vi "send samples.vi"(6 "sample valid before CFO":bool, 7 "use before CFO":bool, 8 "channels before CFO":T1, 9 "packet start":bool, 10 "sample valid after CFO":bool, 11 "channels after CFO":T1) -> ()   [LabVIEW 2020]
uses:
  <vilib>/rvi/interface/RandomDataEmulation/niFpgaRandomDataHandleErrors.vi
  <vilib>/rvi/DataTransferAndStorage/Container/XNode/niFpgaContainer.xnode
  <vilib>/rvi/interface/RandomDataEmulation/nirviRandomDataFpgaReadWriteTemplate.vi
panel:
  out "Imag":fxp<+/-,16,3>
  out "Real":fxp<+/-,16,3>
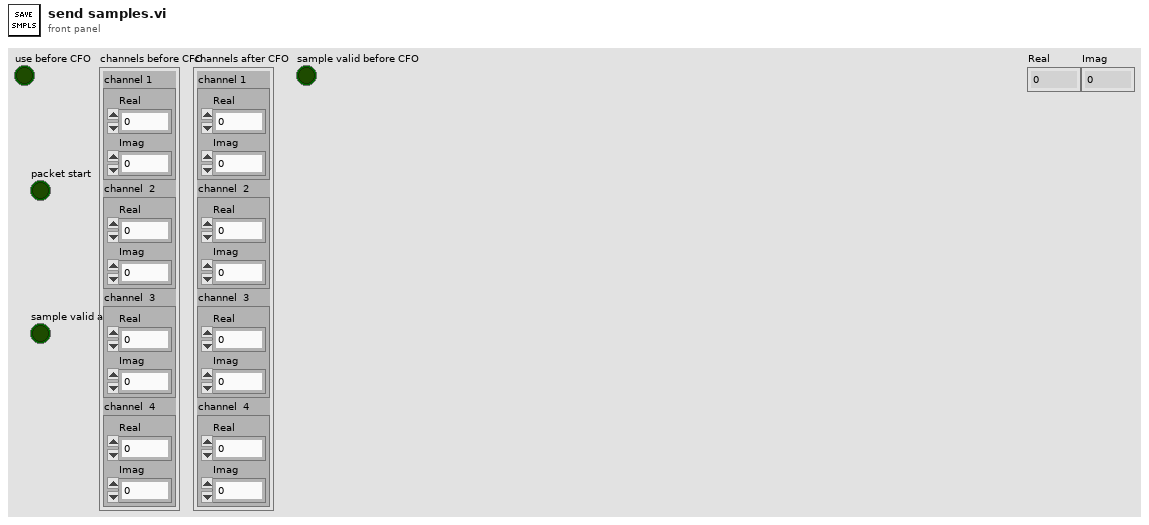
[diagram p1: front panel]
types:
  T1 = cluster{"channel 1 ":cluster{"Real":fxp<+/-,16,3>, "Imag":fxp<+/-,16,3>}, "channel  2":cluster{"Real":fxp<+/-,16,3>, "Imag":fxp<+/-,16,3>}, "channel  3":cluster{"Real":fxp<+/-,16,3>, "Imag":fxp<+/-,16,3>}, "channel  4":cluster{"Real":fxp<+/-,16,3>, "Imag":fxp<+/-,16,3>}}
  T2 = cluster{"Real":fxp<+/-,16,3>, "Imag":fxp<+/-,16,3>}
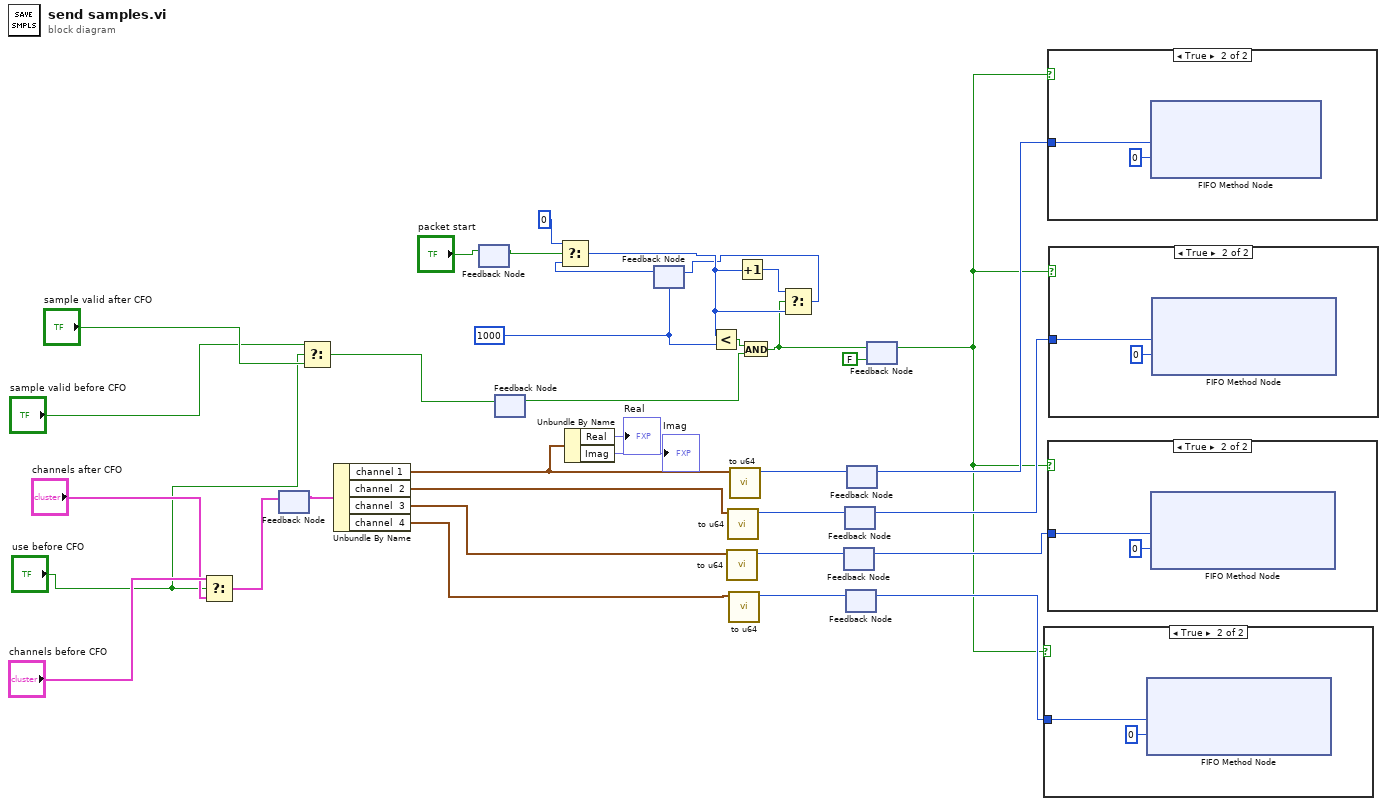
[diagram p0: block diagram]
diagram:
  w25 = u32 1000 ("samples num")
  n1 = Select(t="channels before CFO", s="use before CFO", f="channels after CFO") -> (s? t:f=w8:T1)
  n2 = feedback #1() -> (w21:T1)  [unwired: 1 in]
  n3 = feedback-in #1(w8) -> ()
  n4 = Select(t="sample valid before CFO", s="use before CFO", f="sample valid after CFO") -> (s? t:f=w4:bool)
  n5 = Unbundle By Name(w21) -> ("channel 1"=w7:T2, "channel  2"=w17:T2, "channel  3"=w16:T2, "channel  4"=w15:T2)
  n6 = feedback #2() -> (w23:bool)  [unwired: 1 in]
  n7 = feedback-in #2("packet start") -> ()
  n8 = feedback #3() -> (w24:bool)  [unwired: 1 in]
  n9 = feedback-in #3(w4) -> ()
  n10 = Unbundle By Name(w7) -> ("Real"=→"Real":fxp<+/-,16,3>, "Imag"=→"Imag":fxp<+/-,16,3>)
  n11 = feedback #4(w25) -> (w35:u32)
  n12 = Select(t=u32 0, s=w23, f=w35) -> (s? t:f=w31:u32)
  n13 = Less?(x=w31, y=w25) -> (x < y?=w27:bool)
  n14 = call "to u64.vi"("channel"=w16) -> ("Numeric"=w19:u64)  [unwired: 10 in]
  n15 = call "to u64.vi"("channel"=w17) -> ("Numeric"=w20:u64)  [unwired: 10 in]
  n16 = call "to u64.vi"("channel"=w15) -> ("Numeric"=w18:u64)  [unwired: 10 in]
  n17 = call "to u64.vi"("channel"=w7) -> ("Numeric"=w33:u64)  [unwired: 10 in]
  n18 = Increment(x=w31) -> (x+1=w30:u32)
  n19 = And(x=w27, y=w24) -> (x .and. y?=w26:bool)
  n20 = Select(t=w30, s=w26, f=w31) -> (s? t:f=w29:u32)
  n21 = feedback-in #4(w29) -> ()
  n22 = feedback #5() -> (w13:u64)  [unwired: 1 in]
  n23 = feedback-in #5(w19) -> ()
  n24 = feedback #6() -> (w14:u64)  [unwired: 1 in]
  n25 = feedback-in #6(w20) -> ()
  n26 = feedback #7() -> (w12:u64)  [unwired: 1 in]
  n27 = feedback-in #7(w18) -> ()
  n28 = feedback #8() -> (w32:u64)  [unwired: 1 in]
  n29 = feedback-in #8(w33) -> ()
  n30 = feedback #9(FALSE) -> (w11:bool)
  n31 = feedback-in #9(w26) -> ()
  n32 = case shown="True" w11 {
    tunnel: w12 -> [_ w36]
    frame False {
    }
    frame True {
      n33 = xnode ("FIFO Method Node")("Element"=w36, "Timeout"=0) -> ()  [unwired: 1 in, 2 out]
    }
  }
  n34 = case shown="True" w11 {
    tunnel: w32 -> [_ w38]
    frame False {
    }
    frame True {
      n35 = xnode ("FIFO Method Node")("Element"=w38, "Timeout"=0) -> ()  [unwired: 1 in, 2 out]
    }
  }
  n36 = case shown="True" w11 {
    tunnel: w13 -> [_ w40]
    frame False {
    }
    frame True {
      n37 = xnode ("FIFO Method Node")("Element"=w40, "Timeout"=0) -> ()  [unwired: 1 in, 2 out]
    }
  }
  n38 = case shown="True" w11 {
    tunnel: w14 -> [_ w42]
    frame False {
    }
    frame True {
      n39 = xnode ("FIFO Method Node")("Element"=w42, "Timeout"=0) -> ()  [unwired: 1 in, 2 out]
    }
  }
